vi "More Sensitive Peak Detector.vi"(9 "PD threshold":dbl=1e-06 format="%.2p", 10 "Smooth points":dbl, 11 "Input XY":cluster{dbl[], dbl[]}(graph)) -> (1 "Amplitudes":dbl[](array[numeric]), 2 "Positions":dbl[](array[numeric]), 3 "Locations":dbl[](array[numeric]))   [LabVIEW 2016]
uses:
  <vilib>/Analysis/NI_AAL_SigProc.lvlib
  <vilib>/Analysis/NI_AALPro.lvlib
panel:
  out "second":cluster{dbl[], dbl[]}(graph)
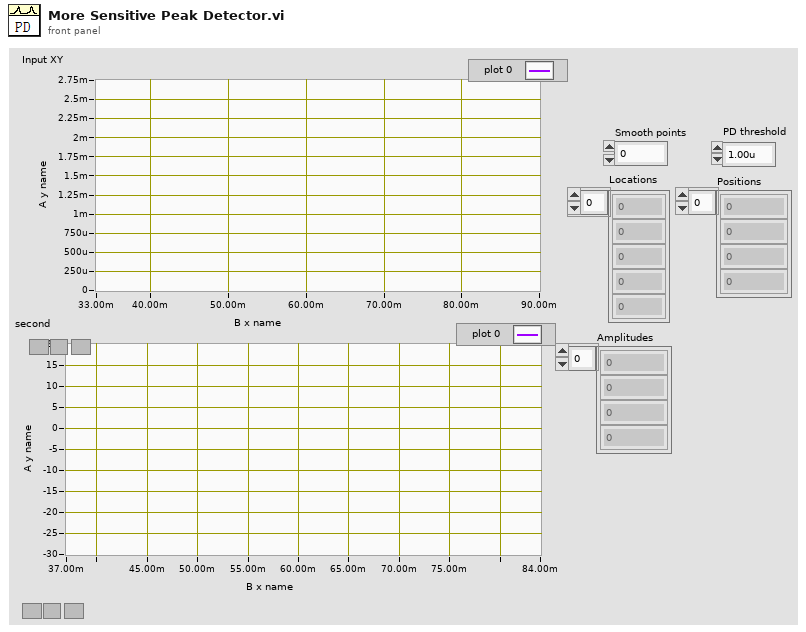
[diagram p1: front panel]
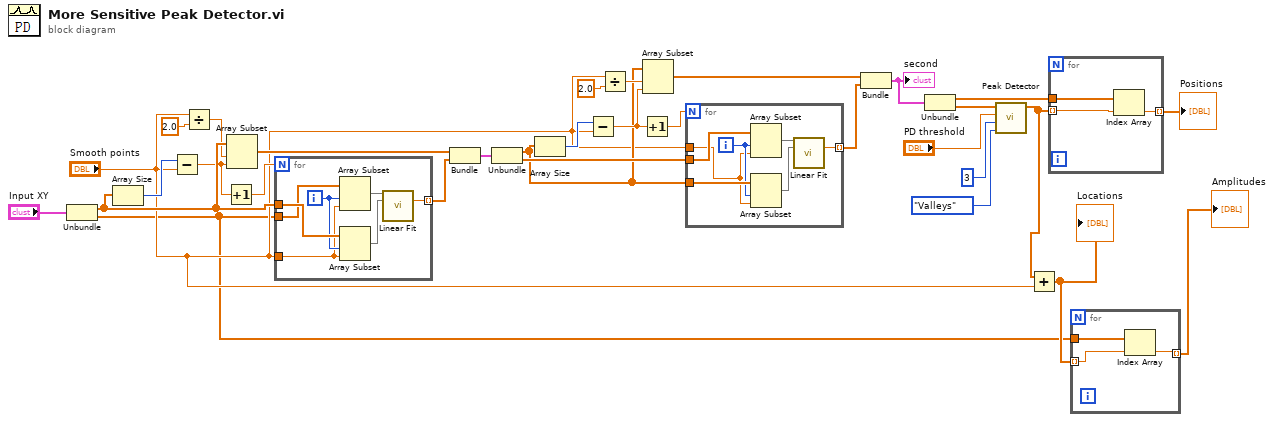
[diagram p0: block diagram]
diagram:
  n1 = Unbundle("Input XY") -> (w23:dbl[], w2:dbl[])
  n2 = Array Size(array=w23) -> (size(s)=w27:i32)
  n3 = Subtract(x=w27, y="Smooth points") -> (x-y=w21:dbl)
  n4 = Divide(x="Smooth points", y=2.0) -> (x/y=w22:dbl)
  n5 = Increment(x=w21) -> (x+1=w26:dbl)
  n6 = Array Subset(array=w23, index=w22, length=w21) -> (w20:dbl[])
  n7 = for {
    N: w26 -> [_]
    tunnel: w23 -> [w38]
    tunnel: w2 -> [w37]
    tunnel: "Smooth points" -> [w35]
    tunnel: [w34] -> w24 mode=indexing
    i -> [w36]
    n8 = Array Subset(array=w37, index=w36, length=w35) -> (w33:dbl[])
    n9 = Array Subset(array=w38, index=w36, length=w35) -> (w32:dbl[])
    n10 = call <vilib>:"Linear Fit.vi"("Y"=w33, "X"=w32) -> ("slope"=w34:dbl)  [unwired: 9 in, 4 out]
  }
  n11 = Bundle(w20, w24) -> (w9:cluster{dbl[], dbl[]})  [unwired: 1 in]
  n12 = Unbundle(w9) -> (w14:dbl[], w15:dbl[])
  n13 = Array Size(array=w14) -> (size(s)=w10:i32)
  n14 = Subtract(x=w10, y="Smooth points") -> (x-y=w17:dbl)
  n15 = Divide(x="Smooth points", y=2.0) -> (x/y=w16:dbl)
  n16 = Increment(x=w17) -> (x+1=w11:dbl)
  n17 = Array Subset(array=w14, index=w16, length=w17) -> (w18:dbl[])
  n18 = for {
    N: w11 -> [_]
    tunnel: w14 -> [w45]
    tunnel: w15 -> [w44]
    tunnel: "Smooth points" -> [w42]
    tunnel: [w41] -> w13 mode=indexing
    i -> [w43]
    n19 = Array Subset(array=w44, index=w43, length=w42) -> (w40:dbl[])
    n20 = Array Subset(array=w45, index=w43, length=w42) -> (w39:dbl[])
    n21 = call <vilib>:"Linear Fit.vi"("Y"=w40, "X"=w39) -> ("slope"=w41:dbl)  [unwired: 9 in, 4 out]
  }
  n22 = Bundle(w18, w13) -> (w8:cluster{dbl[], dbl[]})  [unwired: 1 in]
  "second" <- w8
  n23 = Unbundle(w8) -> (w7:dbl[], w6:dbl[])
  n24 = call <vilib>:"Peak Detector.vi"("peaks/valleys"=enum32{"Peaks", "Valleys"}."Valleys" ("peaks/valleys 2"), "width"=3 ("PD width"), "threshold"="PD threshold", "X"=w6) -> ("Locations"=w5:dbl[])  [unwired: 3 in, 4 out]
  n25 = Add(x=w5, y="Smooth points") -> (x+y=w3:dbl[])
  "Locations" <- w3
  n26 = for {
    tunnel: w7 -> [w48]
    tunnel: w5 -> [w46] mode=indexing
    tunnel: [w47] -> w31 mode=indexing
    n27 = Index Array(array=w48, index=w46) -> (element=w47:dbl)
  }
  "Positions" <- w31
  n28 = for {
    tunnel: w3 -> [w50] mode=indexing
    tunnel: w2 -> [w51]
    tunnel: [w49] -> w1 mode=indexing
    n29 = Index Array(array=w51, index=w50) -> (element=w49:dbl)
  }
  "Amplitudes" <- w1
